vi "Initialize FPGA FIFOs.vi"(8 "error in (no error)":errorcluster, 11 "FGPA Ref":T1) -> (0 "error out":errorcluster, 3 "FGPA Ref":T1)   [LabVIEW 2020]
uses:
  RIG-SPECIFIC FILES/FPGA Refs/FPGA Ref.ctl
  <vilib>/Utility/error.llb/Error Cluster From Error Code.vi
  <vilib>/rvi/interface/common/niFpgaWaitOnOcc.vi
  <vilib>/rvi/interface/nirviMethod/nirviMethod.xnode
  <vilib>/rvi/errors/niLvFpgaMergeErrorWithErrorCode.vi
  <vilib>/FPGAPlugInAG/Dynamic/niLvFpga_StopFifo_Dynamic.vi
  <vilib>/FPGAPlugInAG/Dynamic/niLvFpga_StartFifo_Dynamic.vi
  <vilib>/FPGAPlugInAG/Dynamic/niLvFpga_ConfigureFifo_Dynamic.vi
panel:
  out "Actual Depth":u32
  out "Actual Depth":u32
  out "Actual Depth 2":u32
  out "Actual Depth":u32
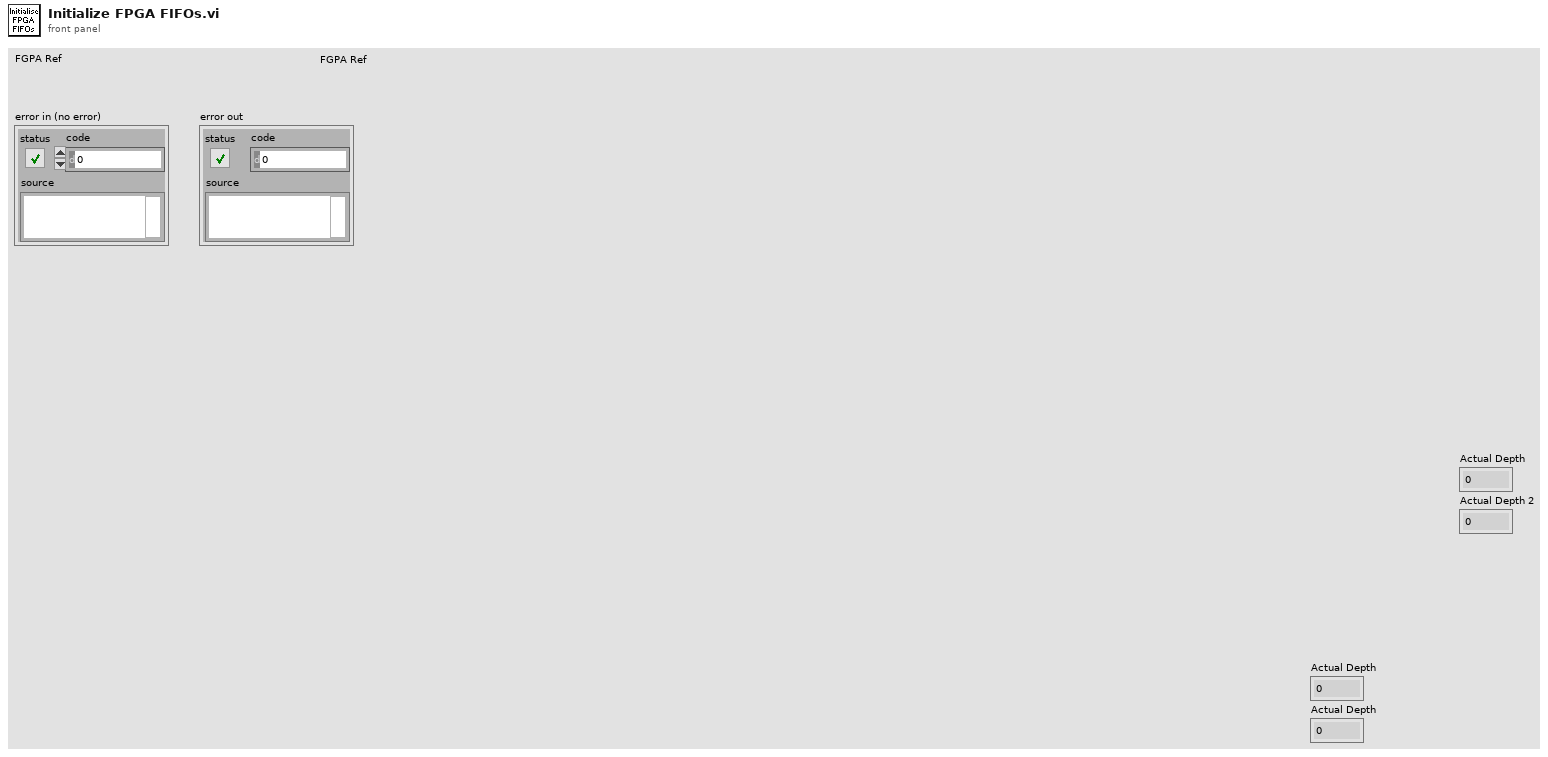
[diagram p1: front panel]
types:
  T1 = typedef "FPGA Ref.ctl" = refnum<k20>
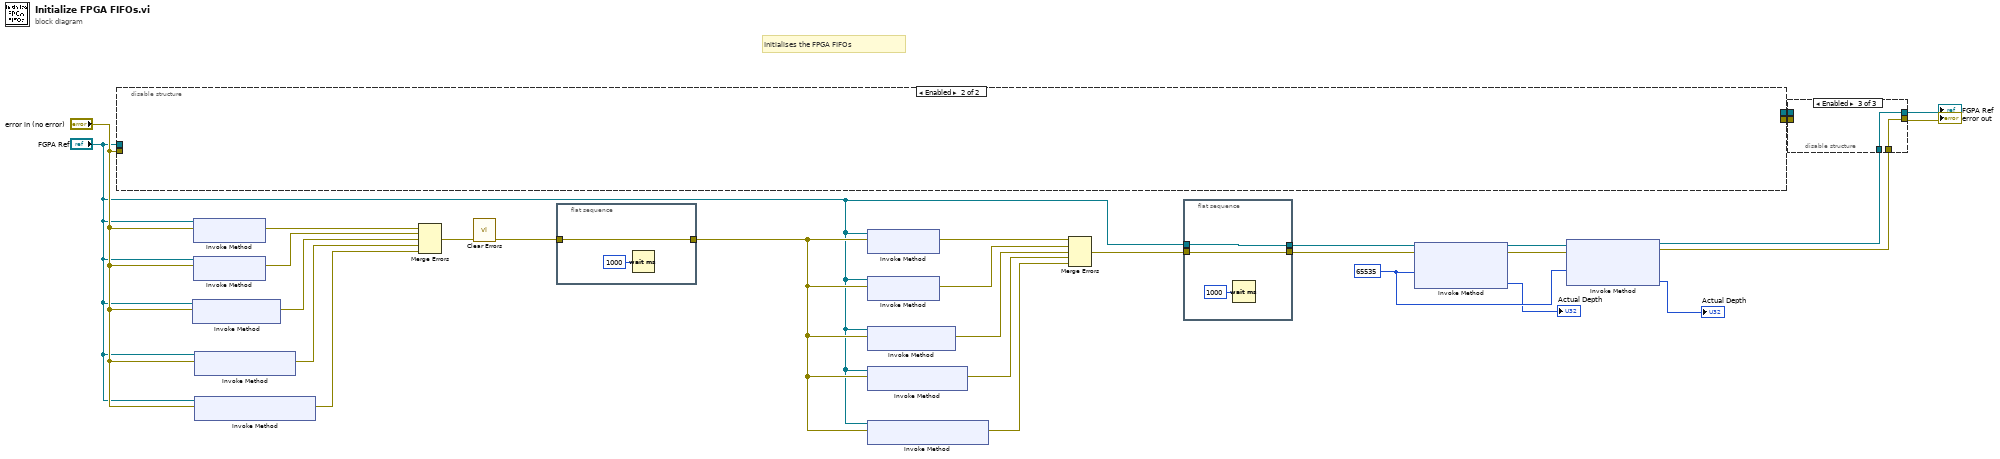
[diagram p0: block diagram]
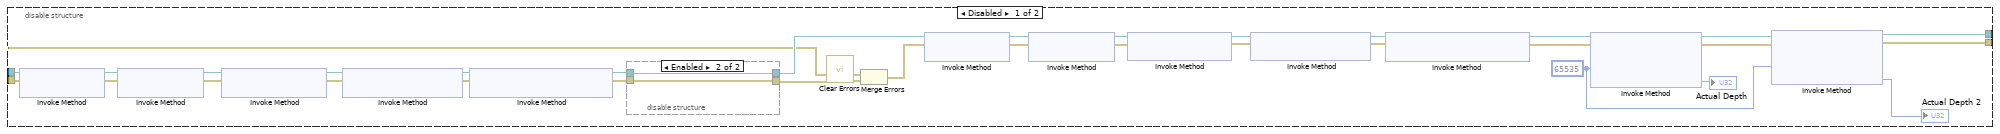
[diagram p2: hidden frame]
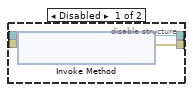
[diagram p3: hidden frame]
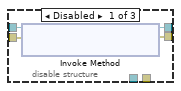
[diagram p4: hidden frame]
diagram:
  w11 = u32 65535 ("Requested Depth")
  # "Initialises the FPGA FIFOs"
  n1 = disable-structure shown="Enabled" {
    disable-tunnel: [w33 _] -> w27
    disable-tunnel: [w32 _] -> w26
    disable-tunnel: "error in (no error)" -> [w31 _]
    disable-tunnel: "FGPA Ref" -> [w30 _]
    frame Disabled {
      w38 = u32 65535 ("Requested Depth")
      n2 = xnode ("Invoke Method")("FPGA VI Reference In"=w30, "error in"=w31) -> ("FPGA VI Reference Out"=w61:T1, "error out"=w59:errorcluster)
      n3 = xnode "Invoke Method"("FPGA VI Reference In"=w61, "error in"=w59) -> ("FPGA VI Reference Out"=w57:T1, "error out"=w56:errorcluster)
      n4 = xnode "Invoke Method"("FPGA VI Reference In"=w57, "error in"=w56) -> ("FPGA VI Reference Out"=w49:T1, "error out"=w48:errorcluster)
      n5 = xnode "Invoke Method"("FPGA VI Reference In"=w49, "error in"=w48) -> ("FPGA VI Reference Out"=w47:T1, "error out"=w46:errorcluster)
      n6 = xnode "Invoke Method"("FPGA VI Reference In"=w47, "error in"=w46) -> ("FPGA VI Reference Out"=w45:T1, "error out"=w44:errorcluster)
      n7 = disable-structure shown="Enabled" {
        disable-tunnel: w45 -> [w66 w68]
        disable-tunnel: w44 -> [w65 w67]
        disable-tunnel: [w64 w67] -> w43
        disable-tunnel: [w63 w68] -> w37
        frame Disabled {
          n8 = xnode "Invoke Method"("FPGA VI Reference In"=w66, "error in"=w65) -> ("FPGA VI Reference Out"=w63:T1, "error out"=w64:errorcluster)
        }
        frame Enabled {
        }
      }
      n9 = call <vilib>:"Clear Errors.vi"("error in (no error)"=w43) -> ("error out"=w60:errorcluster)  [unwired: 5 in, 1 out]
      n10 = Merge Errors(w31, w60) -> (w36:errorcluster)
      n11 = xnode ("Invoke Method")("FPGA VI Reference In"=w37, "error in"=w36) -> ("FPGA VI Reference Out"=w62:T1, "error out"=w58:errorcluster)
      n12 = xnode "Invoke Method"("FPGA VI Reference In"=w62, "error in"=w58) -> ("FPGA VI Reference Out"=w54:T1, "error out"=w55:errorcluster)
      n13 = xnode "Invoke Method"("FPGA VI Reference In"=w54, "error in"=w55) -> ("FPGA VI Reference Out"=w53:T1, "error out"=w52:errorcluster)
      n14 = xnode "Invoke Method"("FPGA VI Reference In"=w53, "error in"=w52) -> ("FPGA VI Reference Out"=w51:T1, "error out"=w50:errorcluster)
      n15 = xnode "Invoke Method"("FPGA VI Reference In"=w51, "error in"=w50) -> ("FPGA VI Reference Out"=w35:T1, "error out"=w34:errorcluster)
      n16 = xnode "Invoke Method"("FPGA VI Reference In"=w35, "error in"=w34, "Requested Depth"=w38) -> ("FPGA VI Reference Out"=w42:T1, "error out"=w41:errorcluster, "Actual Depth"=→"Actual Depth":u32)
      n17 = xnode "Invoke Method"("FPGA VI Reference In"=w42, "error in"=w41, "Requested Depth"=w38) -> ("FPGA VI Reference Out"=w33:T1, "error out"=w32:errorcluster, "Actual Depth"=→"Actual Depth 2":u32)
    }
    frame Enabled {
    }
  }
  n18 = xnode "Invoke Method"("FPGA VI Reference In"="FGPA Ref", "error in"="error in (no error)") -> ("error out"=w22:errorcluster)  [unwired: 1 out]
  n19 = xnode ("Invoke Method")("FPGA VI Reference In"="FGPA Ref", "error in"="error in (no error)") -> ("error out"=w24:errorcluster)  [unwired: 1 out]
  n20 = xnode "Invoke Method"("FPGA VI Reference In"="FGPA Ref", "error in"="error in (no error)") -> ("error out"=w23:errorcluster)  [unwired: 1 out]
  n21 = xnode "Invoke Method"("FPGA VI Reference In"="FGPA Ref", "error in"="error in (no error)") -> ("error out"=w21:errorcluster)  [unwired: 1 out]
  n22 = xnode "Invoke Method"("FPGA VI Reference In"="FGPA Ref", "error in"="error in (no error)") -> ("error out"=w20:errorcluster)  [unwired: 1 out]
  n23 = Merge Errors(w24, w23, w22, w21, w20) -> (w19:errorcluster)
  n24 = call <vilib>:"Clear Errors.vi"("error in (no error)"=w19) -> ("error out"=w18:errorcluster)  [unwired: 5 in, 1 out]
  n25 = flat-sequence {
    tunnel: w18 -> [w69]
    tunnel: [w69] -> w17
    frame #0 {
      n26 = Wait (ms)(milliseconds to wait=u32 1000) -> ()  [unwired: 1 out]
    }
  }
  n27 = xnode ("Invoke Method")("FPGA VI Reference In"="FGPA Ref", "error in"=w17) -> ("error out"=w16:errorcluster)  [unwired: 1 out]
  n28 = xnode "Invoke Method"("FPGA VI Reference In"="FGPA Ref", "error in"=w17) -> ("error out"=w15:errorcluster)  [unwired: 1 out]
  n29 = xnode "Invoke Method"("FPGA VI Reference In"="FGPA Ref", "error in"=w17) -> ("error out"=w14:errorcluster)  [unwired: 1 out]
  n30 = xnode "Invoke Method"("FPGA VI Reference In"="FGPA Ref", "error in"=w17) -> ("error out"=w13:errorcluster)  [unwired: 1 out]
  n31 = xnode "Invoke Method"("FPGA VI Reference In"="FGPA Ref", "error in"=w17) -> ("error out"=w12:errorcluster)  [unwired: 1 out]
  n32 = Merge Errors(w16, w15, w14, w13, w12) -> (w2:errorcluster)
  n33 = flat-sequence {
    tunnel: "FGPA Ref" -> [w73]
    tunnel: [w73] -> w3
    tunnel: w2 -> [w72]
    tunnel: [w72] -> w1
    frame #0 {
      n34 = Wait (ms)(milliseconds to wait=u32 1000) -> ()  [unwired: 1 out]
    }
  }
  n35 = xnode "Invoke Method"("FPGA VI Reference In"=w3, "error in"=w1, "Requested Depth"=w11) -> ("FPGA VI Reference Out"=w7:T1, "error out"=w8:errorcluster, "Actual Depth"=→"Actual Depth":u32)
  n36 = xnode "Invoke Method"("FPGA VI Reference In"=w7, "error in"=w8, "Requested Depth"=w11) -> ("FPGA VI Reference Out"=w6:T1, "error out"=w5:errorcluster, "Actual Depth"=→"Actual Depth":u32)
  n37 = disable-structure shown="Enabled" {
    disable-tunnel: w26 -> [w77 w78 _]
    disable-tunnel: w27 -> [w76 w79 _]
    disable-tunnel: [w75 w79 w81] -> w29
    disable-tunnel: [w74 w78 w80] -> w28
    disable-tunnel: w6 -> [_ _ w81]
    disable-tunnel: w5 -> [_ _ w80]
    frame Disabled {
      n38 = xnode "Invoke Method"("FPGA VI Reference In"=w76, "error in"=w77) -> ("FPGA VI Reference Out"=w75:T1, "error out"=w74:errorcluster)
    }
    frame Disabled {
    }
    frame Enabled {
    }
  }
  "error out" <- w28
  "FGPA Ref" <- w29
